vi "testTelPacketsSentFromTcpServer.vi"(8 "error in (no error)":errorcluster) -> (0 "error out":errorcluster)   [LabVIEW 2018]
uses:
  <vilib>/addons/_JKI Toolkits/Caraya/classes/Assert/Assert Equal Value_Variant.vi
  <vilib>/addons/_JKI Toolkits/Caraya/classes/Test/Test.lvclass
  src/TcpServer/TcpServer.lvclass
  <vilib>/addons/_JKI Toolkits/Caraya/classes/Assert/Assert.lvclass
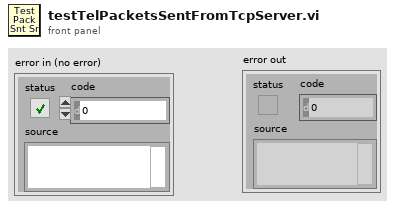
[diagram p1: front panel]
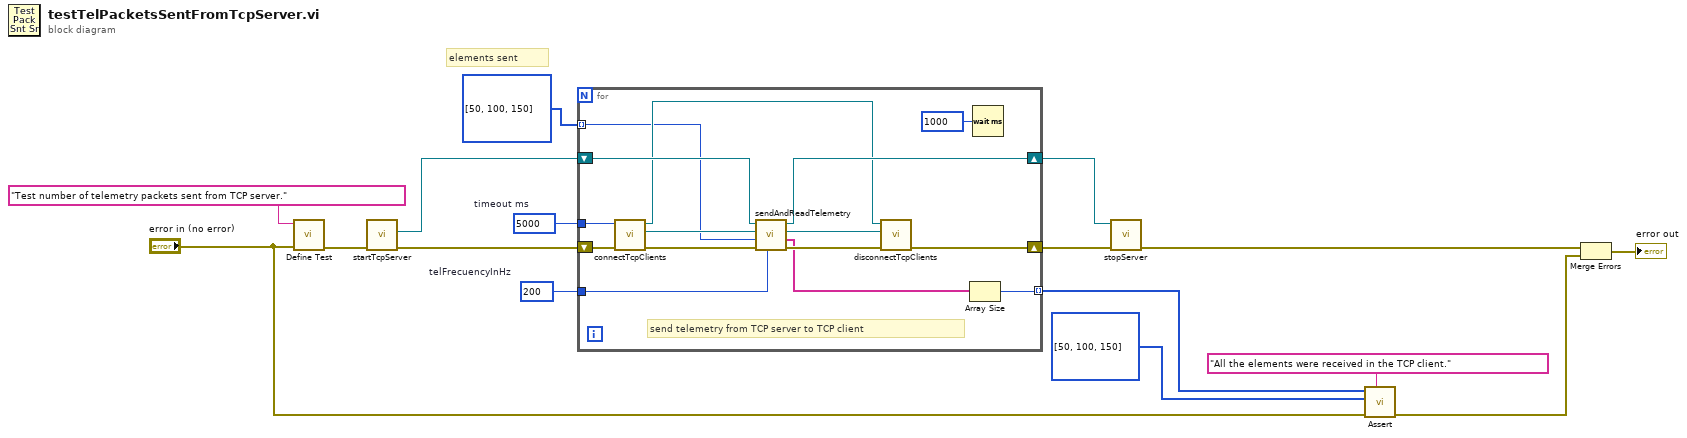
[diagram p0: block diagram]
diagram:
  w1 = u32 200  # telFrecuencyInHz
  w5 = 5000  # timeout ms
  # "elements sent"
  n1 = call <vilib>:"Define Test.vi"("error in (no error)"="error in (no error)", "Label (VI Title)"="Test number of telemetry packets sent from TCP server.") -> ("error out"=w15:errorcluster)  [unwired: 9 in]
  n2 = call "startTcpServer.vi"("error in (no error)"=w15) -> ("error out"=w4:errorcluster, "TcpServer out"=w7:refnum<class "TcpServer.lvclass">)  [unwired: 8 in, 1 out]
  n3 = for {
    shift-right: [w30] -> w14
    shift-left: w4 -> [w31]
    shift-right: [w26] -> w12
    shift-left: w7 -> [w29]
    tunnel: i32[] [50, 100, 150] -> [w22] mode=indexing
    tunnel: w5 -> [w23]
    tunnel: [w18] -> w2 mode=indexing
    tunnel: w1 -> [w17]
    # "send telemetry from TCP server to TCP client"
    n4 = call "connectTcpClients.vi"("error in (no error)"=w31, "timeout ms"=w23) -> ("error out"=w21:errorcluster, "tel connection ID out"=w28:refnum<k5>, "cmd connection ID out"=w25:refnum<k5>)  [unwired: 7 in]
    n5 = call "sendAndReadTelemetry.vi"("telFrecuencyInHz (10)"=w17, "error in (no error)"=w21, "numPackets (50)"=w22, "tel connection in"=w28, "TcpServer out"=w29) -> ("error out"=w20:errorcluster, "telemetry received"=w19:string[], "tel connection out"=w27:refnum<k5>, "tcpServer out"=w26:refnum<class "TcpServer.lvclass">)  [unwired: 3 in]
    n6 = call "disconnectTcpClients.vi"("error in (no error)"=w20, "tel connection ID in"=w27, "cmd connection ID in"=w25) -> ("error out"=w30:errorcluster)  [unwired: 8 in]
    n7 = Array Size(array=w19) -> (size(s)=w18:i32)
    n8 = Wait (ms)(milliseconds to wait=u32 1000) -> ()  [unwired: 1 out]
  }
  n9 = call "stopServer.vi"("error in (no error)"=w14, "tcpServer in"=w12) -> ("error out"=w13:errorcluster)  [unwired: 8 in, 1 out]
  n10 = call-poly <vilib>:"Assert.vi"("Label"="All the elements were received in the TCP client.", "error in (no error)"="error in (no error)", "Y"=i32[] [50, 100, 150], "X"=w2) -> ("error out"=w9:errorcluster)  [unwired: 7 in]
  n11 = Merge Errors(w13, w9) -> (→"error out":errorcluster)
